vi "Test Bed.vi"(0 "Data":i32(listbox)=-1) -> ()   [LabVIEW 2019]
uses:
  <vilib>/Utility/traverseref.llb/VI Scripting - Traverse.lvlib
  <vilib>/Utility/traverseref.llb/TRef TravTarget.ctl
  <vilib>/Utility/miscctls.llb/LVMapReplaceAction.ctl
  controls/Map Key.ctl
  MVA Message Mapper.lvlib
  controls/Datum Endpoint.ctl
  controls/Message Map.ctl
  support/Format Into String Test/Format Into String.lvclass
  support/Build Array Test/Build Array.lvclass
  support/MVA Comms/MVA Comms VI Instance.lvclass
  C:/git/MVA Bus Message Mapper/Source/support/Traversal Algorithm/Node Test.lvclass
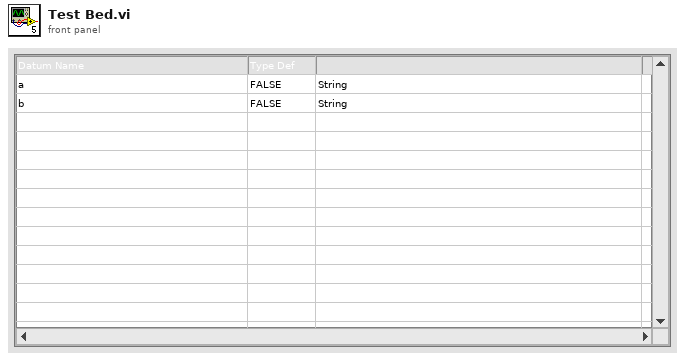
[diagram p1: front panel]
types:
  T1 = typedef "MVA Message Mapper.lvlib/Message Map.ctl" = map{T2, cluster{"Broadcasters":set{T3}, "Receivers":set{T3}}}
  T2 = typedef "MVA Message Mapper.lvlib/Map Key.ctl" = cluster{"Datum Name":string, "Value is TypeDef":bool, "Type String":string}
  T3 = typedef "MVA Message Mapper.lvlib/Datum Endpoint.ctl" = cluster{"Callng VI":path, "Bus VI Name":string, "Source UID":i32, "Sink UID":i32, "Owning Class":string}
  T4 = typedef "TRef TravTarget.ctl" = enum16{"FP", "BD", "Other"}
  T5 = typedef "MVA Message Mapper.lvlib/Set Value.ctl" = cluster{"Callng VI":path, "Bus VI Name":string, "Source UID":i32, "Sink UID":i32, "Owning Class":string}
  T6 = typedef "LVMapReplaceAction.ctl" = enum32{"Modify Entry only if found", "Add or Modify Entry", "Delete Entry"}
  T7 = cluster{"Broadcasters":set{T3}, "Receivers":set{T3}}
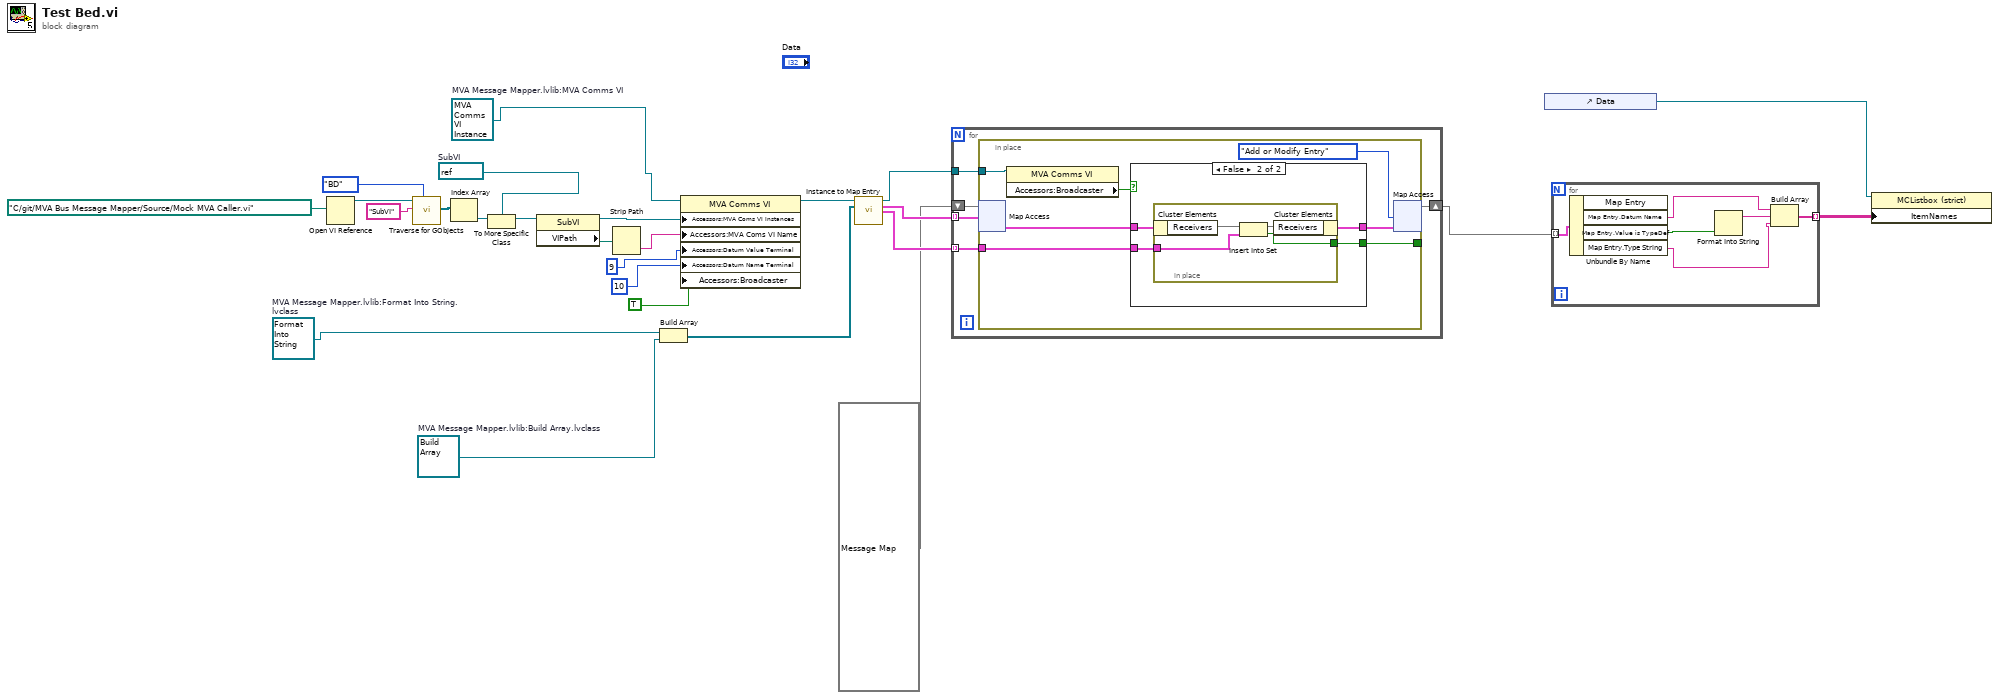
[diagram p0: block diagram]
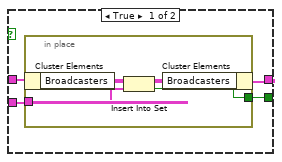
[diagram p2: hidden frame]
diagram:
  w1 = refnum<class "Format Into String.lvclass"> refnum  # MVA Message Mapper.lvlib:Format Into String.lvclass
  w2 = refnum<class "MVA Comms VI Instance.lvclass"> refnum  # MVA Message Mapper.lvlib:MVA Comms VI
  w3 = refnum<class "Build Array.lvclass"> refnum  # MVA Message Mapper.lvlib:Build Array.lvclass
  w21 = refnum<vi> refnum  # SubVI
  n1 = Open VI Reference(vi path=path "C:/git/MVA Bus Message Mapper/Source/Mock MVA Caller.vi") -> (vi reference=w15:refnum<vi>)  [unwired: 5 in, 1 out]
  n2 = call <vilib>:"Traverse for GObjects.vi"("Traverse Target"=TRef_TravTarget."BD", "Class Name"="SubVI", "VI Refnum"=w15) -> ("References"=w24:refnum<vi>[])  [unwired: 5 in, 3 out]
  n3 = Index Array(array=w24) -> (element=w22:refnum<vi>)  [unwired: 1 in]
  n4 = To More Specific Class(target class=w21, reference=w22) -> (specific class reference=w23:refnum<vi>)  [unwired: 1 in, 1 out]
  n5 = property class="SubVI"(reference=w23) -> (reference out=w6:refnum<vi>, "VIPath"=w5:path)  [unwired: 1 in, 1 out]
  n6 = Strip Path(path=w5) -> (name=w19:string)  [unwired: 1 out]
  n7 = Build Array(w1, w3) -> (w4:refnum<class "Node Test.lvclass">[])
  n8 = property class="MVA Comms VI"(reference=w2, "Accessors:MVA Coms VI Instances"=w6, "Accessors:MVA Coms VI Name"=w19, "Accessors:Datum Value Terminal"=9 ("Datum Value Terminal"), "Accessors:Datum Name Terminal"=10 ("Datum Name Terminal"), "Accessors:Broadcaster"=TRUE ("Broadcaster")) -> (reference out=w26:refnum<class "MVA Comms VI Instance.lvclass">)  [unwired: 1 in, 1 out]
  n9 = call-dynamic "Instance to Map Entry.vi"("MVA Comms VI in"=w26, "Node Tests"=w4) -> ("MVA Comms VI out"=w14:refnum<class "MVA Comms VI Instance.lvclass">, "Map Key"=w12:T2[], "Array"=w11:T5[])  [unwired: 10 in, 1 out]
  n10 = for {
    tunnel: w12 -> [w31] mode=indexing
    tunnel: w11 -> [w30] mode=indexing
    tunnel: w14 -> [w29]
    shift-right: [w28] -> w8
    shift-left: T1 {} ("Message Map") -> [w27]
    n11 = in-place {
      in-place-border: w30 -> [w35]
      in-place-border: w29 -> [w34]
      in-place-border: [w32] -> _
      n12 = in-place-map #1(w27, w31) -> (w38:T7)  [unwired: 1 in, 1 out]
      n13 = property class="MVA Comms VI"(reference=w34) -> ("Accessors:Broadcaster"=w33:bool)  [unwired: 1 in, 2 out]
      n14 = case shown="False" w33 {
        tunnel: w38 -> [w42 w50]
        tunnel: [w41 w49] -> w37
        tunnel: w35 -> [w40 w48]
        tunnel: [w39 w47] -> w32
        frame True {
          n15 = in-place {
            in-place-border: w40 -> [w44]
            in-place-border: [w43] -> w39
            n16 = in-place-cluster #2(w42) -> ("Broadcasters"=w46:set{T3})
            n17 = Insert Into Set(10:w44, 11:w46) -> (2:w43:bool, 3:w45:set{T3})
            n18 = in-place-cluster #2("Broadcasters"=w45) -> (w41:T7)
          }
        }
        frame False {
          n19 = in-place {
            in-place-border: w48 -> [w52]
            in-place-border: [w51] -> w47
            n20 = in-place-cluster #3(w50) -> ("Receivers"=w53:set{T3})
            n21 = Insert Into Set(10:w52, 11:w53) -> (2:w51:bool, 3:w54:set{T3})
            n22 = in-place-cluster #3("Receivers"=w54) -> (w49:T7)
          }
        }
      }
      n23 = in-place-map #1(w37, LVMapReplaceAction."Add or Modify Entry" ("action")) -> (w28:T1)  [unwired: 2 out]
    }
  }
  n24 = control-ref of="Data"() -> (w7:refnum<vi>)
  n25 = for {
    tunnel: w8 -> [w56] mode=indexing
    tunnel: [w59] -> w9 mode=indexing
    n26 = Unbundle By Name(w56) -> ("Map Entry.Datum Name"=w57:string, "Map Entry.Value is TypeDef"=w60:bool, "Map Entry.Type String"=w55:string)  [unwired: 1 out]
    n27 = Format Into String(w60) -> (resulting string=w58:string)  [unwired: 3 in, 1 out]
    n28 = Build Array(w57, w58, w55) -> (w59:string[])
  }
  n29 = property class="MCListbox (strict)"(reference=w7, "ItemNames"=w9) -> ()  [unwired: 1 in, 2 out]
